vi "Globals.vi"() -> ()   [LabVIEW 2018]
panel:
  in  "Panel Routine Running":bool
  in  "Cancel Panel Routine":bool
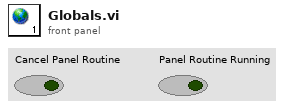
[diagram p1: front panel]
diagram:
